vi "p1.vi"() -> ()   [LabVIEW 2021, in "d17.lvlib"]
uses:
  d17.lvlib
  762ca777-7960-48ca-8045-cc442cda8779.vi
  <vilib>/Comparison/Less/Less Functor/Less Functor.lvclass
  AOC/AOC.lvlib
panel:
  out "shape count":u64=2022
  in  "max shapes":u64=2022
  out "XY Graph":cluster{cluster{"x":i32, "y":i32}[]}[](graph)=[{[{"x"=2, "y"=3168}, {"x"=3, "y"=3168}, {"x"=4, "y"=3168}, {"x"=2, "y"=3169}, {"x"=4, "y"=3169}, {"x"=2, "y"=3170}, {"x"=4, "y"=3170}, {"x"=2, "y"=3171}, {"x"=2, "y"=3172}, {"x"=2, "y"=3173}, {"x"=3, "y"=3173}, {"x"=4, "y"=3173}, {"x"=5, "y"=3173}, {"x"=0, "y"=3174}, {"x"=1, "y"=3174}, {"x"=2, "y"=3174}, {"x"=5, "y"=3174}, {"x"=1, "y"=3175}, {"x"=2, "y"=3175}, {"x"=4, "y"=3175}, {"x"=5, "y"=3175}, {"x"=6, "y"=3175}, {"x"=1, "y"=3176}, {"x"=2, "y"=3176}, {"x"=5, "y"=3176}, {"x"=1, "y"=3177}, {"x"=2, "y"=3177}, {"x"=3, "y"=3177}, {"x"=1, "y"=3178}, {"x"=2, "y"=3178}, {"x"=3, "y"=3178}, {"x"=2, "y"=3179}, {"x"=3, "y"=3179}, {"x"=4, "y"=3179}, {"x"=5, "y"=3179}, {"x"=2, "y"=3180}, {"x"=4, "y"=3180}, {"x"=5, "y"=3180}, {"x"=1, "y"=3181}, {"x"=2, "y"=3181}, {"x"=3, "y"=3181}, {"x"=4, "y"=3181}, {"x"=5, "y"=3181}, {"x"=2, "y"=3182}, {"x"=3, "y"=3182}, {"x"=0, "y"=3183}, {"x"=1, "y"=3183}, {"x"=2, "y"=3183}, {"x"=3, "y"=3183}, {"x"=2, "y"=3184}, {"x"=3, "y"=3184}, {"x"=2, "y"=3185}, {"x"=3, "y"=3185}, {"x"=2, "y"=3186}, {"x"=3, "y"=3186}, {"x"=4, "y"=3186}, {"x"=5, "y"=3186}, {"x"=3, "y"=3187}, {"x"=2, "y"=3188}, {"x"=3, "y"=3188}, {"x"=4, "y"=3188}, {"x"=0, "y"=3189}, {"x"=1, "y"=3189}, {"x"=2, "y"=3189}, {"x"=3, "y"=3189}, {"x"=2, "y"=3190}, {"x"=2, "y"=3191}, {"x"=2, "y"=3192}, {"x"=2, "y"=3193}, {"x"=2, "y"=3194}, {"x"=2, "y"=3195}, {"x"=2, "y"=3196}, {"x"=3, "y"=3196}, {"x"=2, "y"=3197}, {"x"=3, "y"=3197}, {"x"=2, "y"=3198}, {"x"=3, "y"=3198}, {"x"=4, "y"=3198}, {"x"=5, "y"=3198}, {"x"=3, "y"=3199}, {"x"=2, "y"=3200}, {"x"=3, "y"=3200}, {"x"=4, "y"=3200}, {"x"=1, "y"=3201}, {"x"=2, "y"=3201}, {"x"=3, "y"=3201}, {"x"=1, "y"=3202}, {"x"=2, "y"=3202}, {"x"=3, "y"=3202}, {"x"=4, "y"=3202}, {"x"=5, "y"=3202}, {"x"=3, "y"=3203}, {"x"=5, "y"=3203}, {"x"=3, "y"=3204}, {"x"=5, "y"=3204}, {"x"=3, "y"=3205}, {"x"=3, "y"=3206}, {"x"=0, "y"=3207}, {"x"=1, "y"=3207}, {"x"=2, "y"=3207}, {"x"=3, "y"=3207}, {"x"=4, "y"=3207}, {"x"=3, "y"=3208}, {"x"=4, "y"=3208}, {"x"=5, "y"=3208}, {"x"=4, "y"=3209}, {"x"=2, "y"=3210}, {"x"=3, "y"=3210}, {"x"=4, "y"=3210}, {"x"=2, "y"=3211}, {"x"=3, "y"=3211}, {"x"=4, "y"=3211}, {"x"=2, "y"=3212}, {"x"=3, "y"=3212}, {"x"=4, "y"=3212}, {"x"=0, "y"=3213}, {"x"=1, "y"=3213}, {"x"=2, "y"=3213}, {"x"=3, "y"=3213}, {"x"=4, "y"=3213}, {"x"=0, "y"=3214}, {"x"=4, "y"=3214}, {"x"=0, "y"=3215}, {"x"=4, "y"=3215}, {"x"=0, "y"=3216}, {"x"=3, "y"=3216}, {"x"=4, "y"=3216}, {"x"=0, "y"=3217}, {"x"=2, "y"=3217}, {"x"=3, "y"=3217}, {"x"=4, "y"=3217}, {"x"=3, "y"=3218}, {"x"=4, "y"=3218}, {"x"=5, "y"=3218}, {"x"=6, "y"=3218}, {"x"=3, "y"=3219}, {"x"=4, "y"=3219}, {"x"=6, "y"=3219}, {"x"=3, "y"=3220}, {"x"=4, "y"=3220}, {"x"=6, "y"=3220}, {"x"=0, "y"=3221}, {"x"=1, "y"=3221}, {"x"=2, "y"=3221}, {"x"=3, "y"=3221}, {"x"=3, "y"=3222}, {"x"=2, "y"=3223}, {"x"=3, "y"=3223}, {"x"=4, "y"=3223}, {"x"=3, "y"=3224}]}]
  in  "Example":string=">>><<><>><<<>><>>><<<>>><<<><<<>><>><<>>"
  in  "Example":bool
  out "height":i64=3224
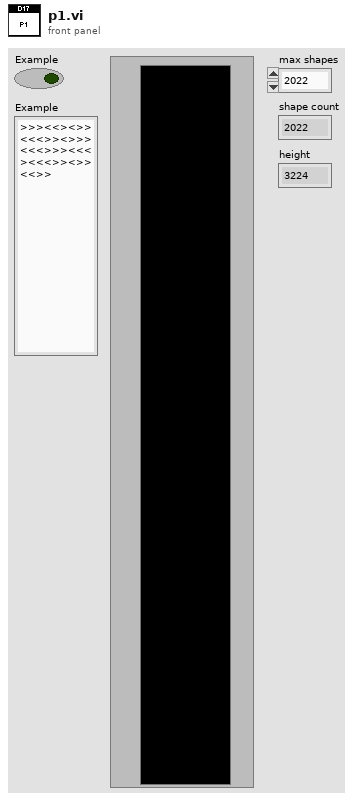
[diagram p1: front panel]
types:
  T1 = cluster{"Co-ordinates":cluster{"x":i8, "y":i8}[]}
  T2 = cluster{"Co-ordinates":cluster{"x":i8, "y":i8}[]}[]
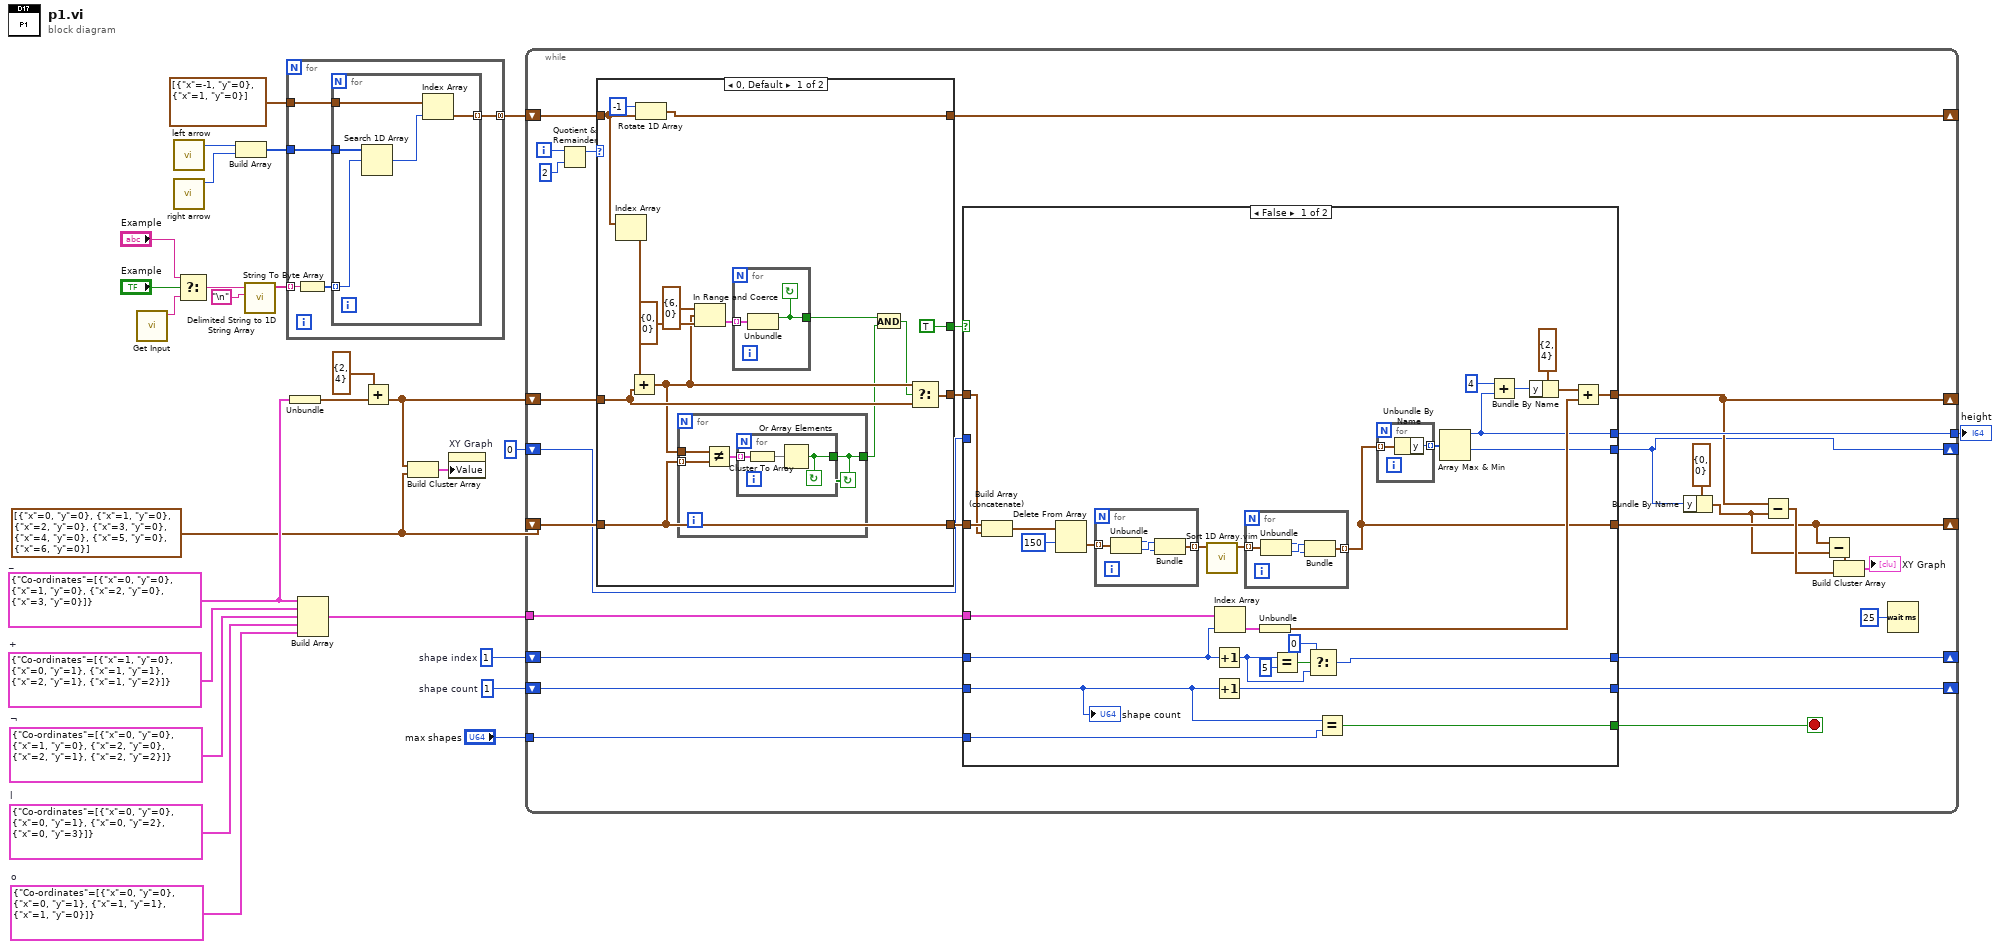
[diagram p0: block diagram]
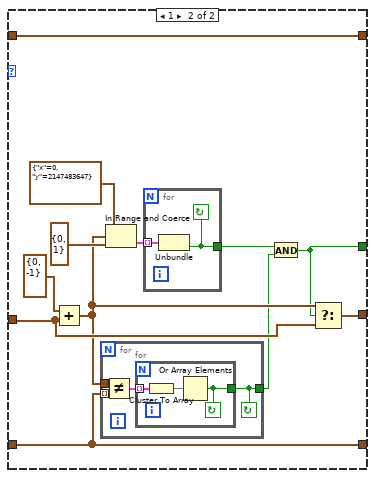
[diagram p3: hidden frame]
diagram:
  w4 = cluster{"x":i32, "y":i32}[] [{"x"=0, "y"=0}, {"x"=1, "y"=0}, {"x"=2, "y"=0}, {"x"=3, "y"=0}, {"x"=4, "y"=0}, {"x"=5, "y"=0}, {"x"=6, "y"=0}]
  w10 = 1  # shape count
  w11 = 1  # shape index
  w13 = T1 {"Co-ordinates"=[{"x"=0, "y"=0}, {"x"=0, "y"=1}, {"x"=1, "y"=1}, {"x"=1, "y"=0}]}  # o
  w14 = T1 {"Co-ordinates"=[{"x"=0, "y"=0}, {"x"=0, "y"=1}, {"x"=0, "y"=2}, {"x"=0, "y"=3}]}  # l
  w15 = T1 {"Co-ordinates"=[{"x"=0, "y"=0}, {"x"=1, "y"=0}, {"x"=2, "y"=0}, {"x"=2, "y"=1}, {"x"=2, "y"=2}]}  # ¬
  w16 = T1 {"Co-ordinates"=[{"x"=1, "y"=0}, {"x"=0, "y"=1}, {"x"=1, "y"=1}, {"x"=2, "y"=1}, {"x"=1, "y"=2}]}  # +
  w8 = T1 {"Co-ordinates"=[{"x"=0, "y"=0}, {"x"=1, "y"=0}, {"x"=2, "y"=0}, {"x"=3, "y"=0}]}  # _
  n1 = call "Get Input.vi"() -> ("Input"=w27:string)  [unwired: 11 in]
  n2 = call "left arrow.vi"() -> ("<"=w20:u8)  [unwired: 11 in]
  n3 = call "right arrow.vi"() -> (">"=w19:u8)  [unwired: 11 in]
  n4 = Select(t="Example", s="Example", f=w27) -> (s? t:f=w26:string)
  n5 = Build Array(w20, w19) -> (w18:u8[])
  n6 = call <vilib>:"Delimited String to 1D String Array.vi"("delimiter"="\n", "delimited string"=w26) -> ("string array"=w22:string[])  [unwired: 9 in]
  n7 = for {
    tunnel: w22 -> [w32] mode=indexing
    tunnel: cluster{"x":i8, "y":i8}[] [{"x"=-1, "y"=0}, {"x"=1, "y"=0}] -> [w29]
    tunnel: w18 -> [w30]
    tunnel: [w28] -> w17 mode=concatenating
    n8 = String To Byte Array(string=w32) -> (unsigned byte array=w31:u8[])
    n9 = for {
      tunnel: w31 -> [w36] mode=indexing
      tunnel: w30 -> [w37]
      tunnel: w29 -> [w35]
      tunnel: [w33] -> w28 mode=indexing
      n10 = Search 1D Array(1D array=w37, element=w36) -> (index of element=w34:i32)  [unwired: 1 in]
      n11 = Index Array(array=w35, index=w34) -> (element=w33:cluster{"x":i8, "y":i8})
    }
  }
  n12 = Unbundle(w8) -> ("Co-ordinates"=w7:cluster{"x":i8, "y":i8}[])
  n13 = Build Array(w8, w16, w15, w14, w13) -> (w12:T2)
  n14 = Add(x=cluster{"x":i8, "y":i8} {"x"=2, "y"=4}, y=w7) -> (x+y=w5:cluster{"x":i8, "y":i8}[])
  n15 = Build Cluster Array(w5, w4) -> (w3:cluster{cluster{"x":i32, "y":i32}[]}[])
  n16 = property on="XY Graph" class="XYGraph (strict)"("Value"=w3) -> ()  [unwired: 2 in, 2 out]
  n17 = while {
    shift-right: [w57] -> _
    shift-left: w17 -> [w65]
    tunnel: w12 -> [w64]
    shift-right: [w62] -> _
    shift-left: w11 -> [w63]
    shift-right: [w44] -> _
    shift-left: w5 -> [w56]
    shift-right: [w48] -> _
    shift-left: w10 -> [w49]
    shift-right: [w40] -> _
    shift-left: w4 -> [w53]
    tunnel: [w51] -> w9
    tunnel: "max shapes" -> [w50]
    shift-right: [w42] -> _
    shift-left: 0 -> [w41]
    i -> [w59]
    stop <- w61 stop-if-true
    n18 = Quotient & Remainder(x=w59, y=2) -> (x-y*floor(x/y)=w60:i32)  [unwired: 1 out]
    n19 = case shown="0, Default" w60 {
      tunnel: w65 -> [w117 w145]
      tunnel: [w123 w145] -> w57
      tunnel: w56 -> [w119 w141]
      tunnel: [w120 w142] -> w55
      tunnel: [TRUE ("y") w136] -> w54
      tunnel: w53 -> [w114 w137]
      tunnel: [w114 w137] -> w52
      frame 0, Default {
        n20 = Index Array(array=w117) -> (element=w112:cluster{"x":i8, "y":i8})  [unwired: 1 in]
        n21 = Add(x=w112, y=w119) -> (x+y=w115:cluster{"x":i32, "y":i32}[])
        n22 = Rotate 1D Array(1:w117, 2:-1 ("n")) -> (0:w123:cluster{"x":i8, "y":i8}[])
        n23 = for {
          tunnel: w115 -> [w126]
          tunnel: w114 -> [w125] mode=indexing
          tunnel: [w128] -> w111
          stop <- w128 continue-if-true
          n24 = Not Equal?(x=w126, y=w125) -> (x != y?=w127:cluster{"x":bool, "y":bool}[])
          n25 = for {
            tunnel: w127 -> [w131] mode=indexing
            tunnel: [w129] -> w128
            stop <- w129 continue-if-true
            n26 = Cluster To Array(cluster=w131) -> (array=w130:bool[])
            n27 = Or Array Elements(Boolean array=w130) -> (logical OR=w129:bool)
          }
        }
        n28 = In Range and Coerce(upper limit=cluster{"x":i8, "y":i8} {"x"=6, "y"=0} ("lower limit"), x=w115, lower limit=cluster{"x":i8, "y":i8} {"x"=0, "y"=0}) -> (In Range?=w110:cluster{"x":bool, "y":bool}[])  [unwired: 1 out]
        n29 = for {
          tunnel: w110 -> [w133] mode=indexing
          tunnel: [w132] -> w118
          stop <- w132 continue-if-true
          n30 = Unbundle(w133) -> ("x"=w132:bool)  [unwired: 1 out]
        }
        n31 = And(x=w118, y=w111) -> (x .and. y?=w113:bool)
        n32 = Select(t=w115, s=w113, f=w119) -> (s? t:f=w120:cluster{"x":i32, "y":i32}[])
      }
      frame 1 {
        n33 = Add(x=cluster{"x":i8, "y":i8} {"x"=0, "y"=-1}, y=w141) -> (x+y=w138:cluster{"x":i32, "y":i32}[])
        n34 = for {
          tunnel: w138 -> [w149]
          tunnel: w137 -> [w148] mode=indexing
          tunnel: [w146] -> w135
          stop <- w146 continue-if-true
          n35 = Not Equal?(x=w149, y=w148) -> (x != y?=w147:cluster{"x":bool, "y":bool}[])
          n36 = for {
            tunnel: w147 -> [w152] mode=indexing
            tunnel: [w150] -> w146
            stop <- w150 continue-if-true
            n37 = Cluster To Array(cluster=w152) -> (array=w151:bool[])
            n38 = Or Array Elements(Boolean array=w151) -> (logical OR=w150:bool)
          }
        }
        n39 = In Range and Coerce(upper limit=cluster{"x":i32, "y":i32} {"x"=0, "y"=2147483647}, x=w138, lower limit=cluster{"x":i8, "y":i8} {"x"=0, "y"=1}) -> (In Range?=w143:cluster{"x":bool, "y":bool}[])  [unwired: 1 out]
        n40 = for {
          tunnel: w143 -> [w154] mode=indexing
          tunnel: [w153] -> w140
          stop <- w153 continue-if-true
          n41 = Unbundle(w154) -> ("y"=w153:bool)  [unwired: 1 out]
        }
        n42 = And(x=w140, y=w135) -> (x .and. y?=w136:bool)
        n43 = Select(t=w138, s=w136, f=w141) -> (s? t:f=w142:cluster{"x":i32, "y":i32}[])
      }
    }
    n44 = case shown="False" w54 {
      tunnel: w64 -> [w94 _]
      tunnel: w63 -> [w92 w109]
      tunnel: [w85 w109] -> w62
      tunnel: [w67 w107] -> w44
      tunnel: w55 -> [w77 w107]
      tunnel: w49 -> [w72 w108]
      tunnel: [w82 w108] -> w48
      tunnel: [w81 _] -> w61
      tunnel: [w68 w106] -> w40
      tunnel: w52 -> [w80 w106]
      tunnel: [w75 _] -> w51
      tunnel: w50 -> [w76 _]
      tunnel: [w66 w105] -> w42
      tunnel: w41 -> [_ w105]
      frame False {
        n45 = Build Array (concatenate)(w80, w77) -> (w74:cluster{"x":i32, "y":i32}[])
        n46 = Delete From Array(array=w74, length=150) -> (deleted portion=w73:cluster{"x":i32, "y":i32}[])  [unwired: 1 in, 1 out]
        n47 = for {
          tunnel: w73 -> [w102] mode=indexing
          tunnel: [w99] -> w70 mode=indexing
          n48 = Unbundle(w102) -> ("x"=w100:i32, "y"=w101:i32)
          n49 = Bundle("y"=w101, "x"=w100) -> (w99:cluster{"y":i32, "x":i32})  [unwired: 1 in]
        }
        n50 = call "Sort 1D Array.vim"("unsorted array"=w70) -> ("sorted array"=w69:cluster{"y":i32, "x":i32}[])  [unwired: 10 in]
        n51 = Increment(x=w92) -> (x+1=w84:i32)
        n52 = Increment(x=w72) -> (x+1=w82:i32)
        n53 = Index Array(array=w94, index=w92) -> (element=w93:T1)
        n54 = for {
          tunnel: w69 -> [w98] mode=indexing
          tunnel: [w95] -> w68 mode=indexing
          n55 = Unbundle(w98) -> ("y"=w96:i32, "x"=w97:i32)
          n56 = Bundle("x"=w97, "y"=w96) -> (w95:cluster{"x":i32, "y":i32})  [unwired: 1 in]
        }
        n57 = Unbundle(w93) -> ("Co-ordinates"=w91:cluster{"x":i8, "y":i8}[])
        n58 = Equal?(x=w84, y=5) -> (x = y?=w86:bool)
        n59 = Select(t=0, s=w86, f=w84) -> (s? t:f=w85:i32)
        n60 = Equal?(x=w72, y=w76) -> (x = y?=w81:bool)
        n61 = for {
          tunnel: w68 -> [w104] mode=indexing
          tunnel: [w103] -> w79 mode=indexing
          n62 = Unbundle By Name(w104) -> ("y"=w103:i32)
        }
        n63 = Array Max & Min(array=w79) -> (max value=w75:i32, min value=w66:i32)  [unwired: 2 out]
        n64 = Add(x=4, y=w75) -> (x+y=w89:i32)
        n65 = Bundle By Name(cluster=cluster{"x":i32, "y":i32} {"x"=2, "y"=4} ("Co-ordinate"), "y"=w89) -> (w88:cluster{"x":i32, "y":i32})
        n66 = Add(x=w88, y=w91) -> (x+y=w67:cluster{"x":i32, "y":i32}[])
        "shape count" <- w72
      }
      frame True {
      }
    }
    n67 = Bundle By Name(cluster=cluster{"x":i32, "y":i32} {"x"=0, "y"=0} ("Co-ordinate"), "y"=w42) -> (w39:cluster{"x":i32, "y":i32})
    n68 = Subtract(x=w44, y=w39) -> (x-y=w43:cluster{"x":i32, "y":i32}[])
    n69 = Subtract(x=w40, y=w39) -> (x-y=w38:cluster{"x":i32, "y":i32}[])
    n70 = Build Cluster Array(w38, w43) -> (→"XY Graph":cluster{cluster{"x":i32, "y":i32}[]}[])
    n71 = Wait (ms)(milliseconds to wait=u32 25) -> ()  [unwired: 1 out]
  }
  "height" <- w9
